vi "Calc_Remaining_Time.vi"(2 "Currently on Row":i32, 3 "Table In":T1[](array[typedef]) {"Carrier_2 Q (l/min)" format="%#.2f"; "Row Duration (mins)" format="%#.1f"; "Row No" min=0; "Trace Gas Concentration (%)" min=0.0 format="%#_4f"; "Carrier_1 Q (l/min)" format="%#.2f"; "Tunnel Speed" format="%#.2f"; "Start X" format="%#.2f"; "Start Y" format="%#.2f"; "Start Z" format="%#.2f"; "End X" format="%#.2f"; "End Y" format="%#.2f"; "End Z" format="%#.2f"; "Averaging time (min)" min=0.0 format="%#.2f"}) -> (0 "Estimated Completion time":string, 1 "Table Out":T1[](array[typedef]) {"Carrier_2 Q (l/min)" format="%#.2f"; "Row Duration (mins)" format="%#.1f"; "Row No" min=0; "Trace Gas Concentration (%)" min=0.0 format="%#_4f"; "Carrier_1 Q (l/min)" format="%#.2f"; "Tunnel Speed" format="%#.2f"; "Start X" format="%#.2f"; "Start Y" format="%#.2f"; "Start Z" format="%#.2f"; "End X" format="%#.2f"; "End Y" format="%#.2f"; "End Z" format="%#.2f"; "Averaging time (min)" min=0.0 format="%#.2f"})   [LabVIEW 2014]
uses:
  Traverse_cluster.ctl
  Spacing.ctl
  Controls/Multi_run_mode.ctl
  Controls/Overhead.ctl
  Globals/Extra_Commands_Global.vi
  Globals/Trav_pos_global.vi
panel:
  # "X           Y            Z"
  # "Start"
  # "End"
  # "X           Y            Z"
  # "Start"
  # "End"
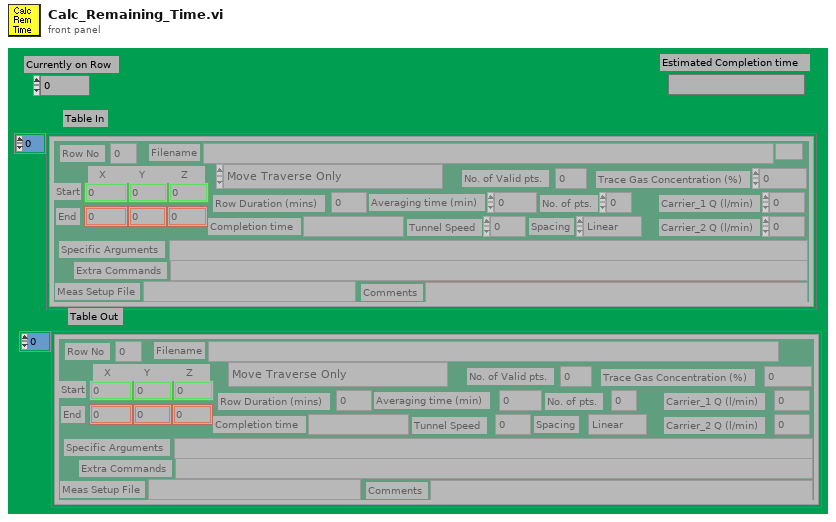
[diagram p1: front panel]
types:
  T1 = typedef "Traverse_cluster.ctl" = cluster{"Start X":sgl, "Start Y":sgl, "Start Z":sgl, "End X":sgl, "End Y":sgl, "End Z":sgl, "No. of pts.":i32, "Spacing":T2, "Filename":path, "Tunnel Speed":dbl, "Averaging time (min)":dbl, "Extra Commands":string, "Carrier_1 Q (l/min)":dbl, "Carrier_2 Q (l/min)":dbl, "Trace Gas Concentration (%)":dbl, "Specific Arguments":string, "Comments":string, "Row No":i32, "Row Type Selector":T3, "Completion time":string, "Row Duration (mins)":dbl, "No. of Valid pts.":i32, "Meas Setup File":string}
  T2 = typedef "Spacing.ctl" = enum16{"Linear", "Log", "Gauss", "Specified", "N/A"}
  T3 = typedef "Multi_run_mode.ctl" = enum16{"Move Traverse Only", "Set Tunnel Speed Only", "Set Source Only", "Set Measurement Conditions", "Single Measurement", "Vertical Profile", "Lateral Profile", "Longitudinal Profile", "Explore Volume", "Multi-Axis Profile", "Auto Calibrate", "Meas Fast FID Bkgnd", "Check Beam Power", "Scanning Valve Measurement", "Run VI Named:", "Set ADAM Ch", "Wait (minutes)", "Send Message", "Synchronize With:", "Fall Back to this Row", "Turn Off Row Repeating", "Blank Row", "Traverse 3D Volume"}
  T4 = typedef "Overhead.ctl" = enum16{"Update total times", "Read Current Overhead", "Re Scale totals to 3 hrs", "Initialise totals to 3hr"}
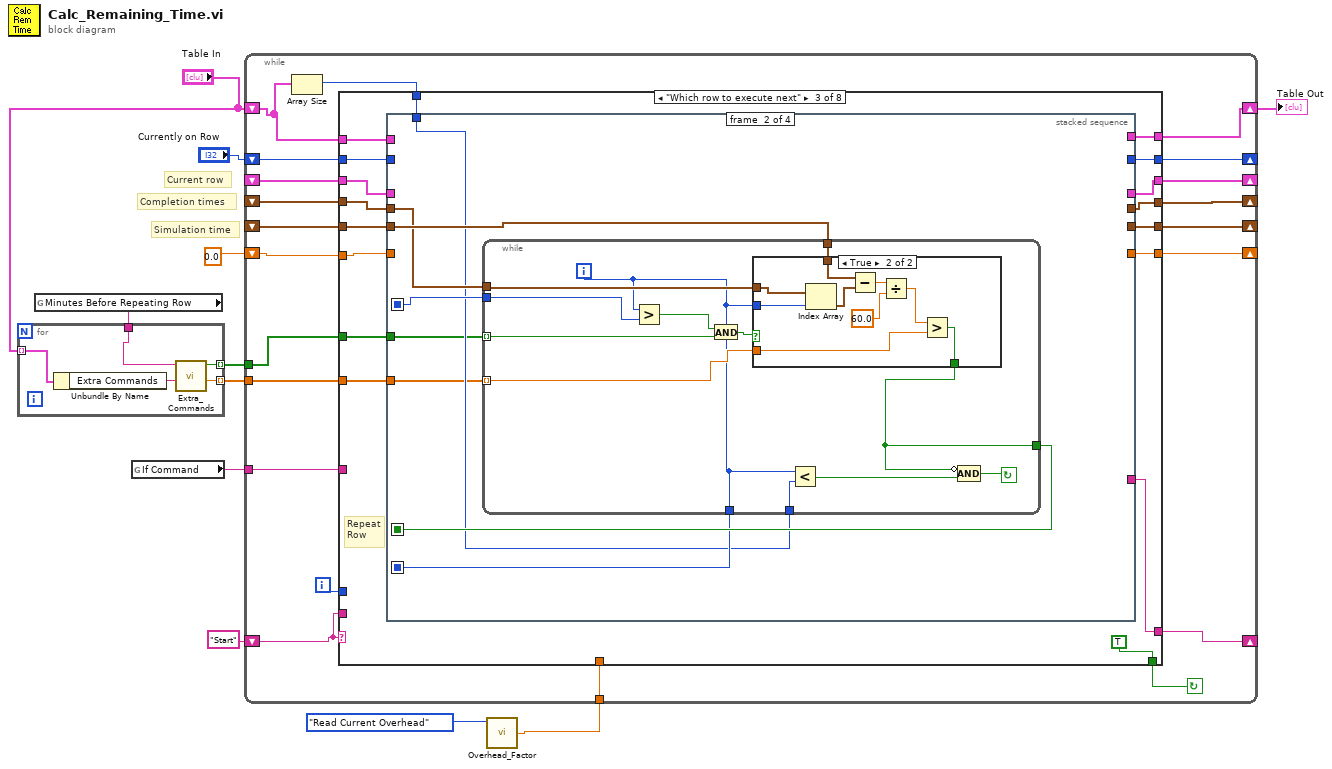
[diagram p0: block diagram]
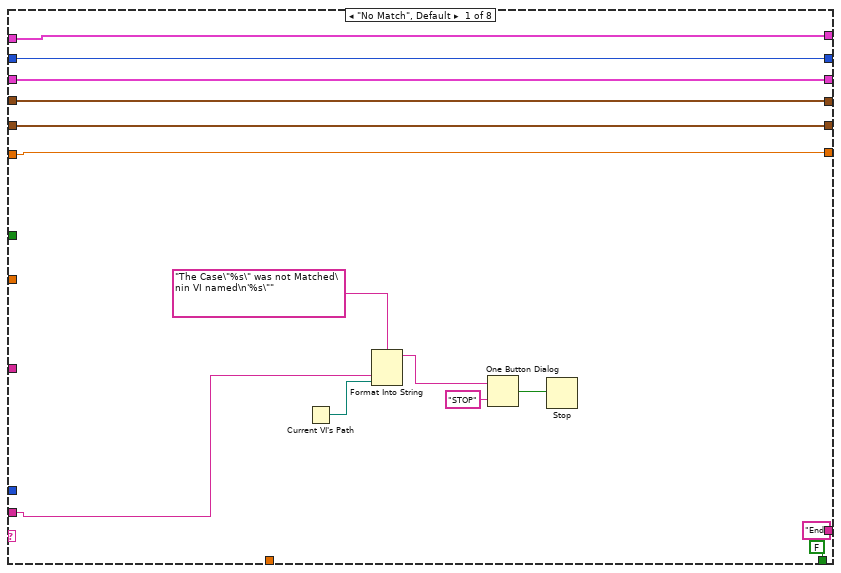
[diagram p2: hidden frame]
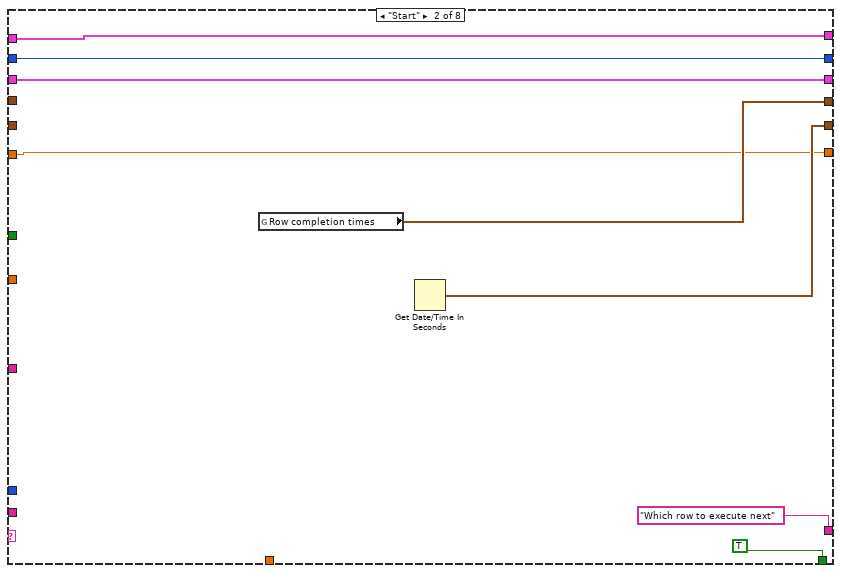
[diagram p3: hidden frame]
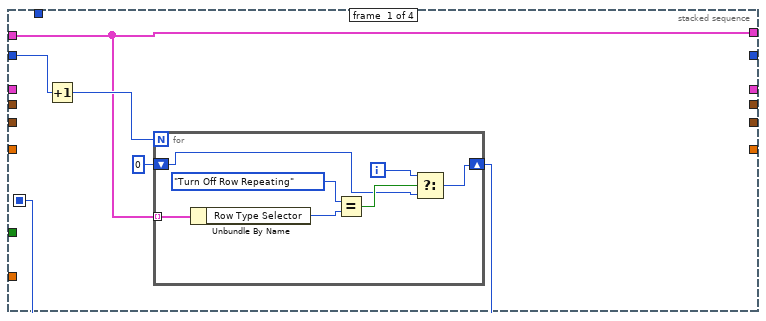
[diagram p4: hidden frame]
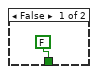
[diagram p5: hidden frame]
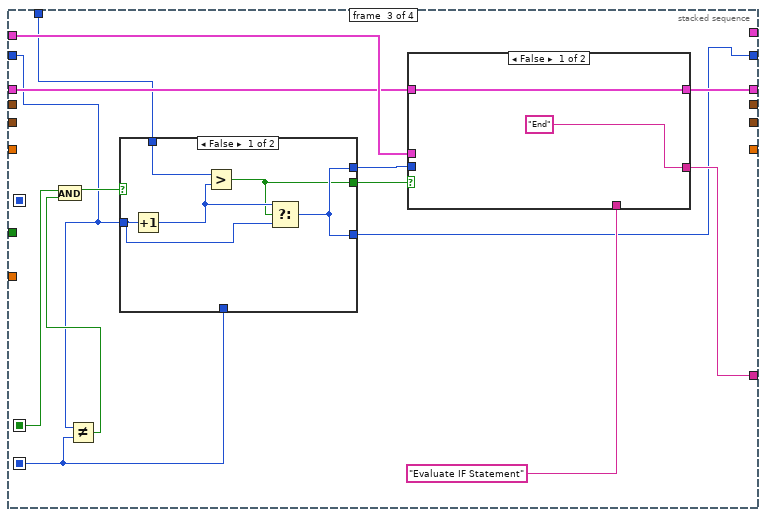
[diagram p6: hidden frame]
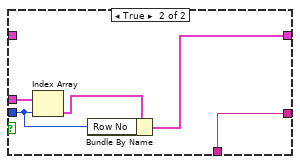
[diagram p7: hidden frame]
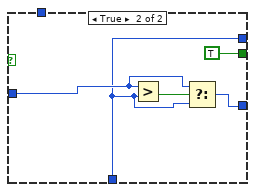
[diagram p8: hidden frame]
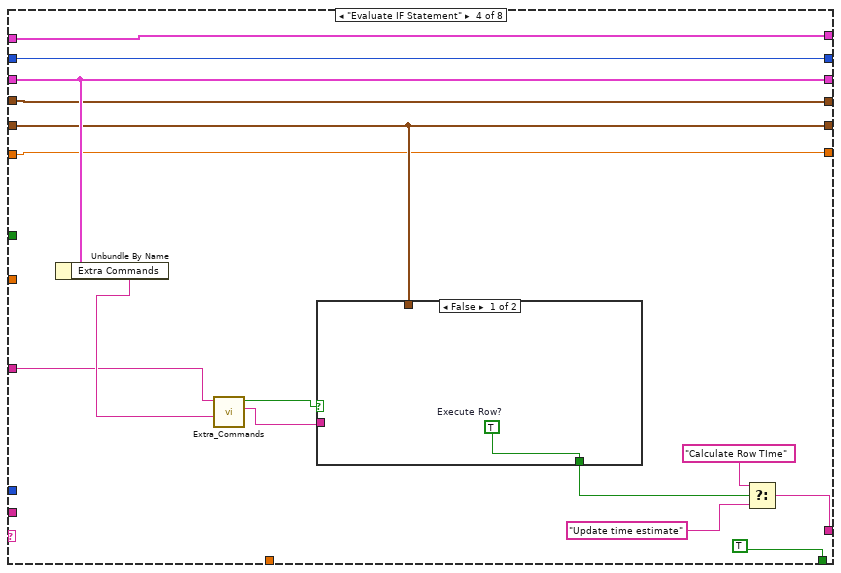
[diagram p10: hidden frame]
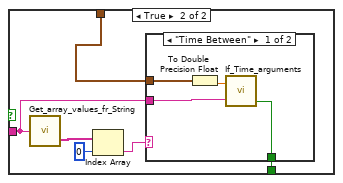
[diagram p11: hidden frame]
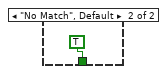
[diagram p12: hidden frame]
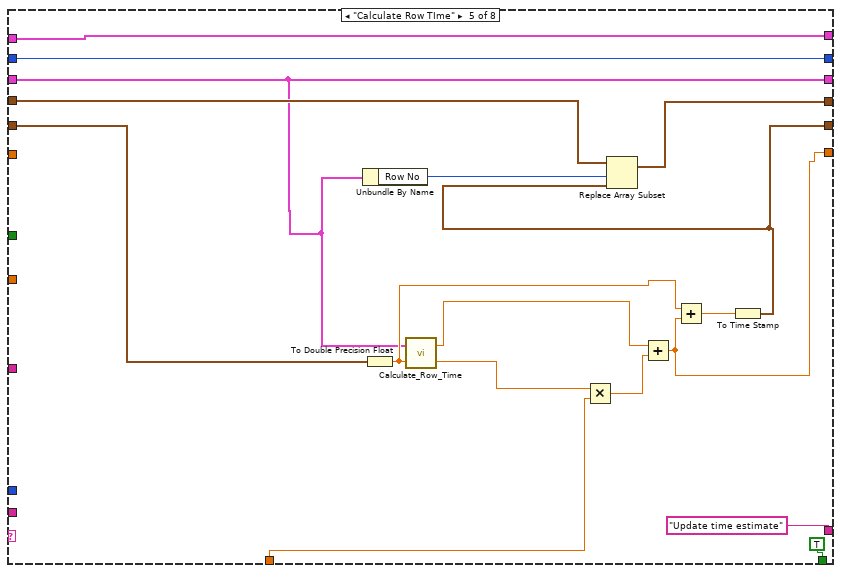
[diagram p13: hidden frame]
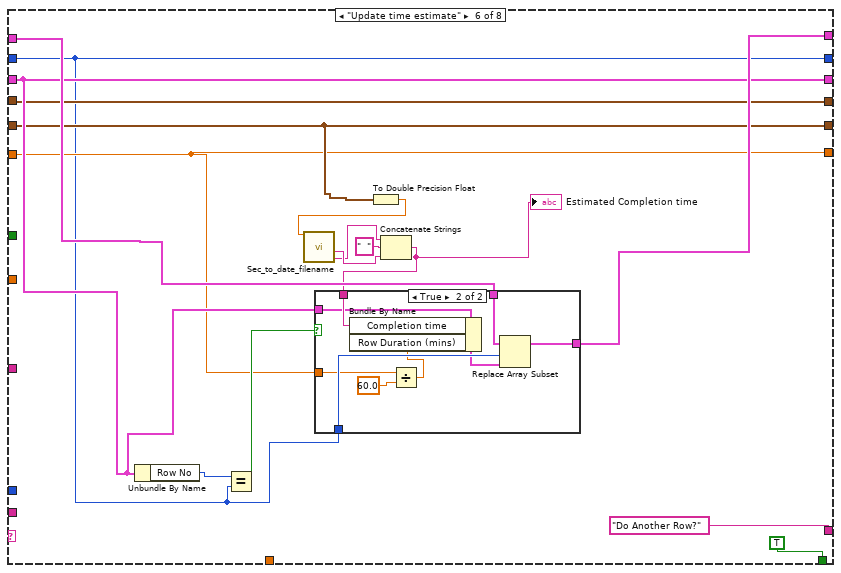
[diagram p14: hidden frame]
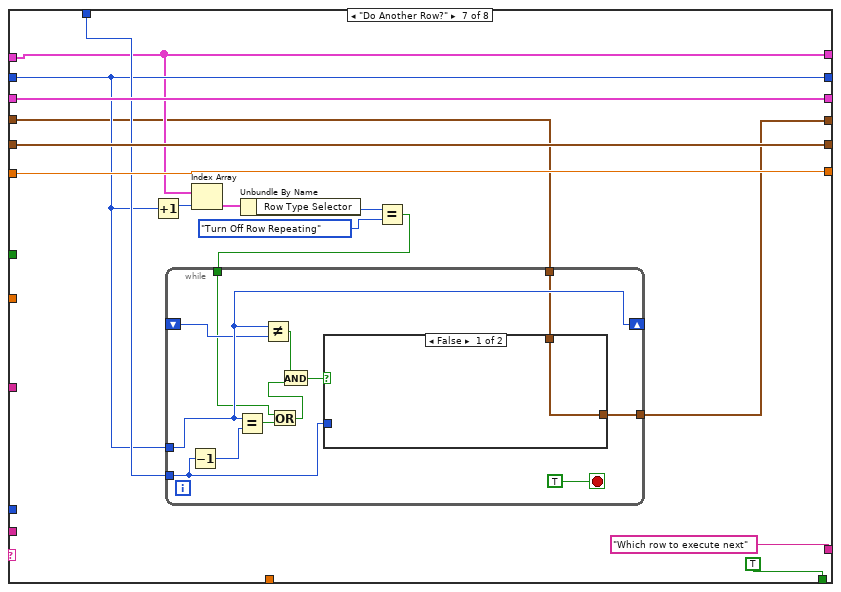
[diagram p16: hidden frame]
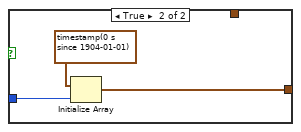
[diagram p17: hidden frame]
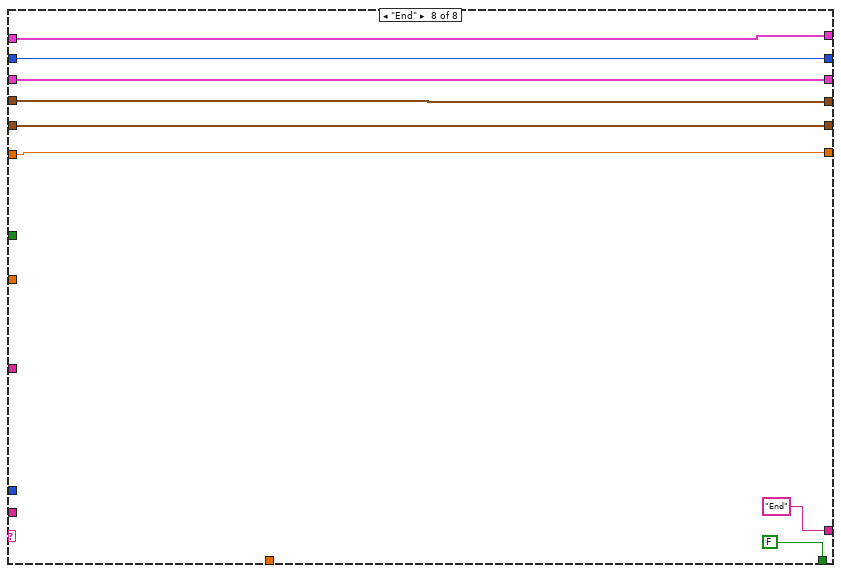
[diagram p18: hidden frame]
diagram:
  # "Simulation time"
  # "Completion times"
  # "Current row"
  n1 = global read "Extra_Commands_Global.vi" "Minutes Before Repeating Row"() -> (w1:string)
  n2 = for {
    tunnel: "Table In" -> [w15] mode=indexing
    tunnel: [w14] -> w3 mode=indexing
    tunnel: [w13] -> w2 mode=indexing
    tunnel: w1 -> [w12]
    n3 = Unbundle By Name(w15) -> ("Extra Commands"=w16:string)
    n4 = call "Extra_Commands.vi"("String to Search"=w16, "Command"=w12) -> ("Numeric Value"=w13:dbl, "Command Found"=w14:bool)  [unwired: 1 in, 3 out]
  }
  n5 = global read "Extra_Commands_Global.vi" "If Command"() -> (w7:string)
  n6 = call "Overhead_Factor.vi"("Mode"=Overhead."Read Current Overhead") -> ("Current Overhead Factor"=w8:dbl)  [unwired: 3 in]
  n7 = while {
    shift-left: "Start" -> [w35]
    shift-right: [w34] -> _
    shift-right: [w32] -> w10
    shift-left: "Table In" -> [w21]
    tunnel: w8 -> [w31]
    shift-right: [w30] -> _
    shift-left: _ -> [w29]
    shift-right: [w25] -> _
    shift-left: _ -> [w26]
    shift-right: [w27] -> _
    shift-left: _ -> [w28]
    shift-right: [w22] -> _
    shift-left: "Currently on Row" -> [w23]
    tunnel: w7 -> [w24]
    shift-right: [w20] -> _
    shift-left: 0.0 ("row Duration") -> [w19]
    tunnel: w3 -> [w18]
    tunnel: w2 -> [w17]
    i -> [w36]
    stop <- w37 continue-if-true
    n8 = Array Size(array=w21) -> (size(s)=w33:i32)
    n9 = case shown="\"Which row to execute next\"" w35 {
      tunnel: [FALSE ("Continue?") TRUE ("Continue?") TRUE ("Continue?") TRUE TRUE TRUE TRUE FALSE] -> w37
      tunnel: w21 -> [w45 w59 w74 w164 w195 w211 w225 w260]
      tunnel: w35 -> [w46 _ _ _ _ _ _ _]
      tunnel: w36 -> [_ _ _ _ _ _ _ _]
      tunnel: ["End" "Which row to execute next" w72 w166 "Update time estimate" "Do Another Row?" "Which row to execute next" "End"] -> w34
      tunnel: w33 -> [_ _ w73 _ _ _ w231 _]
      tunnel: [w45 w59 w75 w164 w195 w210 w225 w260] -> w32
      tunnel: w31 -> [_ _ _ _ w188 _ _ _]
      tunnel: [w42 w54 w71 w156 w182 w201 w235 w258] -> w30
      tunnel: w29 -> [w42 w54 w70 w156 w182 w201 w235 w258]
      tunnel: w28 -> [w39 _ w69 w154 w183 w199 w234 w256]
      tunnel: [w39 w56 w64 w154 w186 w199 w234 w256] -> w27
      tunnel: w26 -> [w40 _ w68 w155 w185 w200 w223 w257]
      tunnel: [w40 w55 w65 w155 w184 w200 w232 w257] -> w25
      tunnel: w24 -> [_ _ _ w158 _ _ _ _]
      tunnel: w23 -> [w41 w53 w67 w157 w181 w197 w226 w255]
      tunnel: [w41 w53 w66 w157 w181 w197 w226 w255] -> w22
      tunnel: [w38 w52 w62 w153 w180 w198 w233 w254] -> w20
      tunnel: w19 -> [w38 w52 w63 w153 _ w198 w233 w254]
      tunnel: w18 -> [_ _ w61 _ _ _ _ _]
      tunnel: w17 -> [_ _ w60 _ _ _ _ _]
      frame "No Match", Default {
        n10 = Current VI's Path() -> (path=w47:path)
        n11 = Format Into String(format string="The Case\"%s\" was not Matched\nin VI named\n'%s\"" ("Format String"), w46, w47) -> (resulting string=w50:string)  [unwired: 2 in, 1 out]
        n12 = One Button Dialog(message=w50, button name ("OK")="STOP") -> (true=w48:bool)
        n13 = Stop(stop? (T)=w48) -> ()
      }
      frame "Start" {
        n14 = global read "Trav_pos_global.vi" "Row completion times"() -> (w55:timestamp[])
        n15 = Get Date/Time In Seconds() -> (seconds since 1Jan1904=w56:timestamp)
      }
      frame "Which row to execute next" {
        # "Repeat\nRow"
        n16 = stacked-sequence {
          seq-local: [_ w96 _ _] -> [_ _ w127 _]
          seq-local: [_ w95 _ _] -> [_ _ w128 _]
          seq-local: [w77 _ _ _] -> [_ w94 _ _]
          tunnel: [w78 _ _ _] -> w75
          tunnel: w74 -> [w78 _ w131 _]
          tunnel: w73 -> [_ w91 w120 _]
          tunnel: [_ _ w129 _] -> w72
          tunnel: [_ _ w123 _] -> w71
          tunnel: w70 -> [_ _ w122 _]
          tunnel: w69 -> [_ w93 _ w151]
          tunnel: w68 -> [_ w92 _ w152]
          tunnel: w67 -> [w81 _ w121 _]
          tunnel: [_ _ w119 _] -> w66
          tunnel: [_ _ _ w152] -> w65
          tunnel: [_ _ _ w151] -> w64
          tunnel: w63 -> [_ _ _ w150]
          tunnel: [_ _ _ w150] -> w62
          tunnel: w61 -> [_ w90 _ _]
          tunnel: w60 -> [_ w89 _ _]
          frame #0 {
            n17 = Increment(x=w81) -> (x+1=w79:i32)
            n18 = for {
              N: w79 -> [_]
              tunnel: w78 -> [w88] mode=indexing
              shift-right: [w85] -> w77
              shift-left: 0 -> [w82]
              i -> [w83]
              n19 = Unbundle By Name(w88) -> ("Row Type Selector"=w87:T3)
              n20 = Equal?(x=Multi_run_mode."Turn Off Row Repeating" ("Row Type Selector"), y=w87) -> (x = y?=w84:bool)
              n21 = Select(t=w83, s=w84, f=w82) -> (s? t:f=w85:i32)
            }
          }
          frame #1 {
            n22 = while {
              tunnel: w92 -> [w108]
              tunnel: w93 -> [w107]
              tunnel: [w102] -> w96
              tunnel: [w99] -> w95
              tunnel: w94 -> [w98]
              tunnel: w91 -> [w103]
              tunnel: w90 -> [w101] mode=indexing
              tunnel: w89 -> [w100] mode=indexing
              i -> [w99]
              stop <- w106 continue-if-true
              n23 = Greater?(x=w99, y=w98) -> (0:w97:bool)
              n24 = And(x=w97, y=w101) -> (x .and. y?=w104:bool)
              n25 = case shown="True" w104 {
                tunnel: w108 -> [_ w114]
                tunnel: w107 -> [_ w115]
                tunnel: w99 -> [_ w113]
                tunnel: w100 -> [_ w111]
                tunnel: [FALSE w110] -> w102
                frame False {
                }
                frame True {
                  n26 = Index Array(array=w114, index=w113) -> (element=w116:timestamp)
                  n27 = Subtract(x=w115, y=w116) -> (x-y=w117:dbl)
                  n28 = Divide(x=w117, y=60.0) -> (x/y=w112:dbl)
                  n29 = Greater?(x=w112, y=w111) -> (0:w110:bool)
                }
              }
              n30 = Less?(x=w99, y=w103) -> (x < y?=w105:bool)
              n31 = Compound Arithmetic op=AND(invert w102, w105) -> (w106:bool)
            }
          }
          frame #2 {
            n32 = Not Equal?(x=w121, y=w128) -> (x != y?=w126:bool)
            n33 = And(x=w127, y=w126) -> (x .and. y?=w125:bool)
            n34 = case shown="False" w125 {
              tunnel: w128 -> [_ w146]
              tunnel: w121 -> [w142 w148]
              tunnel: [w141 w147] -> w119
              tunnel: [w141 w146] -> w132
              tunnel: w120 -> [w144 _]
              tunnel: [w140 TRUE] -> w130
              frame False {
                n35 = Increment(x=w142) -> (x+1=w143:i32)
                n36 = Greater?(x=w144, y=w143) -> (0:w140:bool)
                n37 = Select(t=w143, s=w140, f=w142) -> (s? t:f=w141:i32)
              }
              frame True {
                n38 = Greater?(x=w148, y=w146) -> (0:w149:bool)
                n39 = Select(t=w148, s=w149, f=w146) -> (s? t:f=w147:i32)
              }
            }
            n40 = case shown="False" w130 {
              tunnel: w132 -> [_ w136]
              tunnel: w131 -> [_ w139]
              tunnel: ["End" w138] -> w129
              tunnel: "Evaluate IF Statement" -> [_ w138]
              tunnel: [w133 w135] -> w123
              tunnel: w122 -> [w133 _]
              frame False {
              }
              frame True {
                n41 = Index Array(array=w139, index=w136) -> (element=w137:T1)
                n42 = Bundle By Name(cluster=w137, "Row No"=w136) -> (w135:T1)
              }
            }
          }
          frame #3 {
          }
        }
      }
      frame "Evaluate IF Statement" {
        n43 = Unbundle By Name(w156) -> ("Extra Commands"=w163:string)
        n44 = call "Extra_Commands.vi"("String to Search"=w163, "Command"=w158) -> ("String Value"=w165:string, "Command Found"=w161:bool)  [unwired: 1 in, 3 out]
        n45 = case shown="False" w161 {
          tunnel: w165 -> [_ w171]
          tunnel: [w168 w170] -> w162
          tunnel: w154 -> [_ w169]
          frame False {
            w168 = TRUE  # Execute Row?
          }
          frame True {
            n46 = call "Get_array_values_fr_String.vi"("String Value"=w171) -> ("String array"=w173:string[])  [unwired: 1 out]
            n47 = Index Array(array=w173, index=0 ("Index")) -> (element=w172:string)
            n48 = case shown="\"Time Between\"" w172 {
              tunnel: w171 -> [w178 _]
              tunnel: [w177 TRUE ("Execute Row?")] -> w170
              tunnel: w169 -> [w175 _]
              frame "Time Between" {
                n49 = To Double Precision Float(number=w175) -> (double precision float=w176:dbl)
                n50 = call "If_Time_arguments.vi"("seconds since 1Jan1904"=w176, "String Value"=w178) -> ("Execute Row?"=w177:bool)  [unwired: 2 out]
              }
              frame "No Match", Default {
              }
            }
          }
        }
        n51 = Select(t="Calculate Row TIme", s=w162, f="Update time estimate") -> (s? t:f=w166:string)
      }
      frame "Calculate Row TIme" {
        n52 = Unbundle By Name(w182) -> ("Row No"=w194:i32)
        n53 = To Double Precision Float(number=w183) -> (double precision float=w191:dbl)
        n54 = call "Calculate_Row_Time.vi"("Row Start Time (Sec Since 1904)"=w191, "Multi Run Row"=w182) -> ("Scalable Time (Sec)"=w189:dbl, "Fixed Time (Sec)"=w192:dbl)
        n55 = Multiply(x=w189, y=w188) -> (x*y=w193:dbl)
        n56 = Add(x=w192, y=w193) -> (x+y=w180:dbl)
        n57 = Add(x=w191, y=w180) -> (x+y=w190:dbl)
        n58 = To Time Stamp(1:w190) -> (0:w186:timestamp)
        n59 = Replace Array Subset(array=w185, new element=w186, index=w194) -> (w184:timestamp[])
      }
      frame "Update time estimate" {
        n60 = Unbundle By Name(w201) -> ("Row No"=w209:i32)
        n61 = Equal?(x=w209, y=w197) -> (x = y?=w208:bool)
        n62 = To Double Precision Float(number=w199) -> (double precision float=w204:dbl)
        n63 = call "Sec_to_date_filename.vi"("seconds"=w204) -> ("Day"=w206:string, "Time"=w205:string)  [unwired: 2 out]
        n64 = Concatenate Strings(w205, "  " ("Substring"), w206) -> (w203:string)
        "Estimated Completion time" <- w203
        n65 = case shown="True" w208 {
          tunnel: w197 -> [_ w222]
          tunnel: w211 -> [w213 w221]
          tunnel: [w213 w219] -> w210
          tunnel: w203 -> [_ w218]
          tunnel: w201 -> [_ w217]
          tunnel: w198 -> [_ w214]
          frame False {
          }
          frame True {
            n66 = Divide(x=w214, y=60.0) -> (x/y=w215:dbl)
            n67 = Bundle By Name(cluster=w217, "Completion time"=w218, "Row Duration (mins)"=w215) -> (w220:T1)
            n68 = Replace Array Subset(array=w221, new element=w220, index=w222) -> (w219:T1[])
          }
        }
      }
      frame "Do Another Row?" {
        n69 = Increment(x=w226) -> (x+1=w229:i32)
        n70 = Index Array(array=w225, index=w229) -> (element=w230:T1)
        n71 = Unbundle By Name(w230) -> ("Row Type Selector"=w227:T3)
        n72 = Equal?(x=w227, y=Multi_run_mode."Turn Off Row Repeating" ("Row Type Selector")) -> (x = y?=w224:bool)
        n73 = while {
          shift-right: [w248] -> _
          shift-left: _ -> [w247]
          tunnel: w231 -> [w244]
          tunnel: w226 -> [w248]
          tunnel: w224 -> [w241]
          tunnel: [w239] -> w232
          tunnel: w223 -> [w238]
          stop <- TRUE stop-if-true
          n74 = Decrement(x=w244) -> (x-1=w249:i32)
          n75 = Equal?(x=w248, y=w249) -> (x = y?=w242:bool)
          n76 = Not Equal?(x=w248, y=w247) -> (x != y?=w246:bool)
          n77 = Or(x=w241, y=w242) -> (x .or. y?=w240:bool)
          n78 = And(x=w246, y=w240) -> (x .and. y?=w245:bool)
          n79 = case shown="False" w245 {
            tunnel: w244 -> [_ w252]
            tunnel: [w250 w251] -> w239
            tunnel: w238 -> [w250 _]
            frame False {
            }
            frame True {
              n80 = Initialize Array(timestamp(0 s since 1904-01-01) ("seconds since 1Jan1904"), w252) -> (w251:timestamp[])
            }
          }
        }
      }
      frame "End" {
      }
    }
  }
  "Table Out" <- w10
